vi "BuildSELECTString.vi"(9 "columns":string[](array[string]), 11 "table":string) -> (2 "select query":string=" ")   [LabVIEW 2019, in "libpqutility.lvlib"]
doc: "creates with table and columns SQL Select String like this:\nSELECT column1, column2, ..., columnN FROM table"
uses:
  libpqutility.lvlib
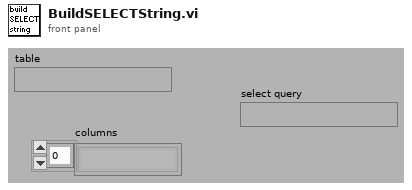
[diagram p1: front panel]
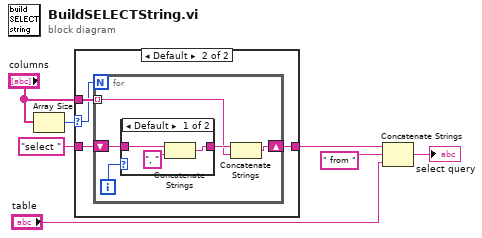
[diagram p0: block diagram]
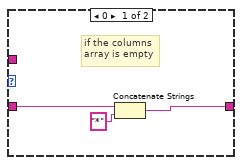
[diagram p2: hidden frame]
diagram:
  n1 = Array Size(array="columns") -> (size(s)=w7:i32)
  n2 = case shown="Default" w7 {
    selector: w7 -> [_ w11]
    tunnel: "columns" -> [_ w14]
    tunnel: [w9 w13] -> w2
    tunnel: "select " ("Substring") -> [w8 w12]
    frame 0 {
      # "if the columns\narray is empty"
      n3 = Concatenate Strings(w8, "*" ("Substring")) -> (w9:string)
    }
    frame Default {
      n4 = for {
        N: w11 -> [_]
        tunnel: w14 -> [w16] mode=indexing
        shift-right: [w15] -> w13
        shift-left: w12 -> [w18]
        i -> [w19]
        n5 = case shown="Default" w19 {
          tunnel: w18 -> [w22 w23]
          tunnel: [w20 w23] -> w17
          frame Default {
            n6 = Concatenate Strings(w22, ", " ("Substring")) -> (w20:string)
          }
          frame 0 {
          }
        }
        n7 = Concatenate Strings(w17, w16) -> (w15:string)
      }
    }
  }
  n8 = Concatenate Strings(w2, " from " ("Substring"), "table") -> (→"select query":string)
